vi "topmostVI.vi"() -> ()   [LabVIEW 2017]
panel:
  out "VI Path":path
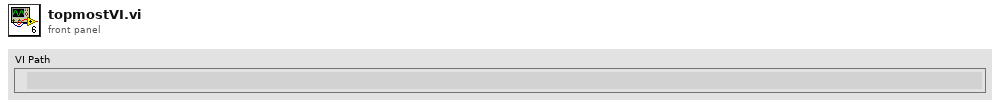
[diagram p1: front panel]
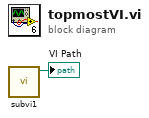
[diagram p0: block diagram]
diagram:
  n1 = call "subvi1.vi"() -> ("VI Path"=→"VI Path":path)  [unwired: 11 in]
